vi "CreateFile_in_a_folder_if_not_exists.vi"(0 "Operator's Name":string, 1 "Data output folder":string="E:\\Ankit\\") -> (2 "filename":string, 3 "String":string, 4 "Path":path, 5 "index":i32)   [LabVIEW 2013]
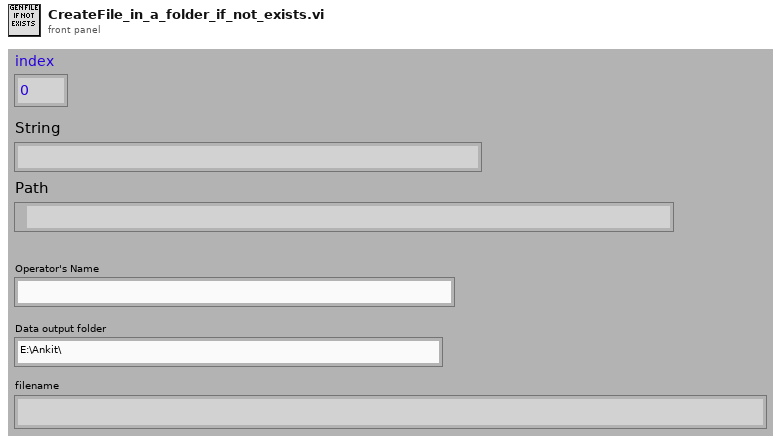
[diagram p1: front panel]
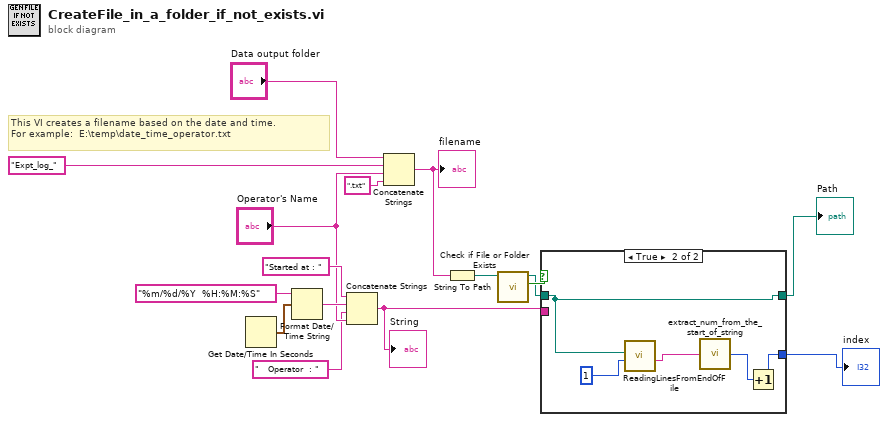
[diagram p0: block diagram]
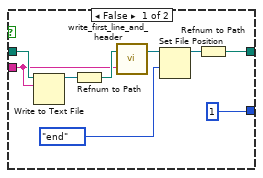
[diagram p2: hidden frame]
diagram:
  # "This VI creates a filename based on the date and time.\nFor example:  E:\\temp\\date_time_operator.txt"
  n1 = Get Date/Time In Seconds() -> (seconds since 1Jan1904=w12:timestamp)
  n2 = Format Date/Time String(time format string (%c)="%m/%d/%Y  %H:%M:%S", seconds (now)=w12) -> (date/time string=w10:string)  [unwired: 1 out]
  n3 = Concatenate Strings("Started at : " ("text"), w10, "   Operator  : " ("text"), "Operator's Name") -> (w3:string)
  "String" <- w3
  n4 = Concatenate Strings("Data output folder", "Expt_log_" ("time format string (%c)"), "Operator's Name", ".txt" ("string")) -> (w16:string)
  "filename" <- w16
  n5 = String To Path(string=w16) -> (path=w6:path)
  n6 = call <vilib>:"Check if File or Folder Exists.vi"("path"=w6) -> ("file or folder exists?"=w5:bool, "dup path"=w4:path)  [unwired: 8 in, 1 out]
  n7 = case shown="True" w5 {
    tunnel: w4 -> [w25 w28]
    tunnel: w3 -> [w22 _]
    tunnel: [w19 w28] -> w2
    tunnel: [1 w26] -> w1
    frame False {
      n8 = Write to Text File(file (use dialog)=w25, text=w22) -> (refnum out=w24:refnum<file>)  [unwired: 1 in, 3 out]
      n9 = Refnum to Path(1:w24) -> (0:w23:path)
      n10 = call "write_first_line_and_header.vi"("first_line"=w22, "Path"=w23) -> ("Byte Stream File out"=w21:refnum<file>)  [unwired: 1 out]
      n11 = Set File Position(refnum=w21, from (0:start)=enum16{"start", "end", "current"}."end") -> (refnum out=w20:refnum<file>)  [unwired: 2 in, 1 out]
      n12 = Refnum to Path(1:w20) -> (0:w19:path)
    }
    frame True {
      n13 = call "ReadingLinesFromEndOfFile.vi"("How Many Rows?"=1, "File Path"=w28) -> ("Selected Rows"=w29:string)  [unwired: 8 in, 1 out]
      n14 = call "extract_num_from_the_start_of_string.vi"("Input String"=w29) -> ("numeric output"=w27:i32)
      n15 = Increment(x=w27) -> (x+1=w26:i32)
    }
  }
  "Path" <- w2
  "index" <- w1
